vi "DiagramDisable.vi"() -> ()   [LabVIEW 2019]
panel:
  out "Numeric":dbl
  in  "num2":dbl
  in  "num1":dbl
  out "y":bool
  in  "b":bool
  in  "a":bool
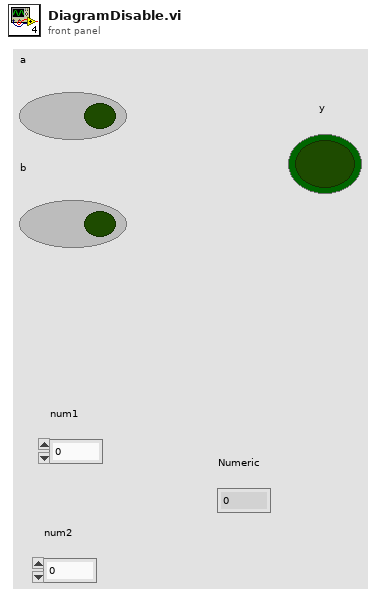
[diagram p1: front panel]
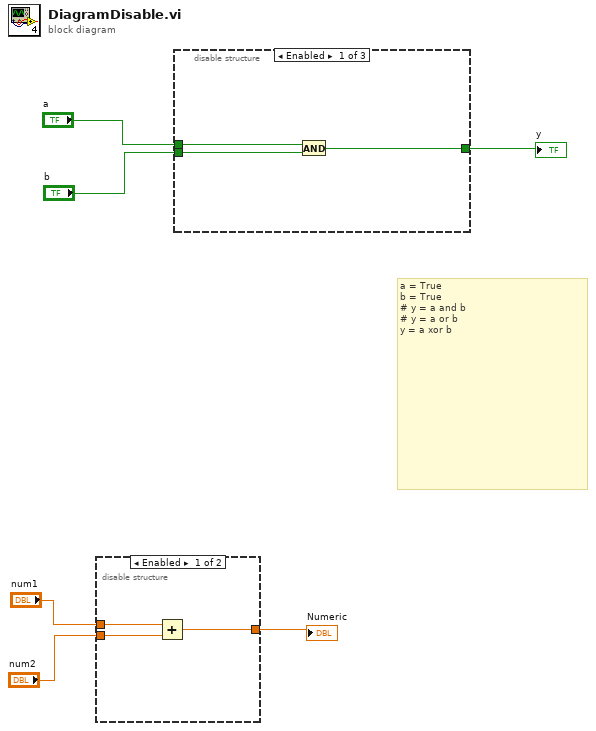
[diagram p0: block diagram]
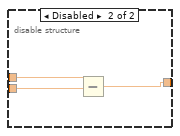
[diagram p2: hidden frame]
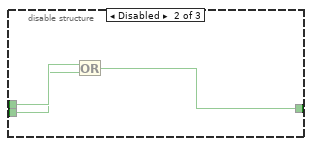
[diagram p3: hidden frame]
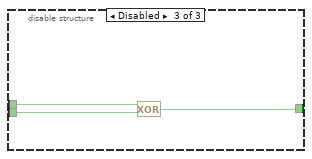
[diagram p4: hidden frame]
diagram:
  # "a = True\nb = True\n# y = a and b\n# y = a or b\ny = a xor b"
  n1 = disable-structure shown="Enabled" {
    disable-tunnel: "num1" -> [w9 w12]
    disable-tunnel: "num2" -> [w8 w11]
    disable-tunnel: [w7 w10] -> w1
    frame Enabled {
      n2 = Add(x=w9, y=w8) -> (x+y=w7:dbl)
    }
    frame Disabled {
      n3 = Subtract(x=w12, y=w11) -> (x-y=w10:dbl)
    }
  }
  "Numeric" <- w1
  n4 = disable-structure shown="Enabled" {
    disable-tunnel: "a" -> [w15 w18 w21]
    disable-tunnel: "b" -> [w14 w17 w20]
    disable-tunnel: [w13 w16 w19] -> w4
    frame Enabled {
      n5 = And(x=w15, y=w14) -> (x .and. y?=w13:bool)
    }
    frame Disabled {
      n6 = Or(x=w18, y=w17) -> (x .or. y?=w16:bool)
    }
    frame Disabled {
      n7 = Exclusive Or(1:w20, 2:w21) -> (0:w19:bool)
    }
  }
  "y" <- w4
